vi "ESC_control.vi"(3 "Mode":T5=enum."Run VI", 5 "Traverse line In":T2={"Start X"=0.0, "Start Y"=0.0, "Start Z"=0.0, "End X"=0.0, "End Y"=0.0, "End Z"=0.0, "No. of pts."=0, "Spacing"=enum."Linear", "Filename"=path "", "Tunnel Speed"=0.0, "Averaging time (min)"=0.0, "Extra Commands"="", "Carrier_1 Q (l/min)"=0.0, "Carrier_2 Q (l/min)"=0.0, "Trace Gas Concentration (%)"=0.0, "Specific Arguments"="Source_Live_Control.vi; 1", "Comments"="", "Row No"=0, "Row Type Selector"=enum."Move Traverse Only", "Completion time"="", "Row Duration (mins)"=0.0, "No. of Valid pts."=0, "Meas Setup File"=""} {"Carrier_2 Q (l/min)" format="%#.2f"; "Row Duration (mins)" format="%#.1f"; "Row No" min=0; "Trace Gas Concentration (%)" min=0.0 format="%#_4f"; "Carrier_1 Q (l/min)" format="%#.2f"; "Tunnel Speed" format="%#.2f"; "Start X" format="%#.2f"; "Start Y" format="%#.2f"; "Start Z" format="%#.2f"; "End X" format="%#.2f"; "End Y" format="%#.2f"; "End Z" format="%#.2f"; "Averaging time (min)" min=0.0 format="%#.2f"}) -> (0 "Error Message":string, 1 "Status":T1, 2 "Traverse line Out":T2={"Start X"=0.0, "Start Y"=0.0, "Start Z"=0.0, "End X"=0.0, "End Y"=0.0, "End Z"=0.0, "No. of pts."=0, "Spacing"=enum."Linear", "Filename"=path "", "Tunnel Speed"=0.0, "Averaging time (min)"=0.0, "Extra Commands"="", "Carrier_1 Q (l/min)"=0.0, "Carrier_2 Q (l/min)"=0.0, "Trace Gas Concentration (%)"=0.0, "Specific Arguments"="Source_Live_Control.vi; 1", "Comments"="", "Row No"=0, "Row Type Selector"=enum."Move Traverse Only", "Completion time"="", "Row Duration (mins)"=0.0, "No. of Valid pts."=0, "Meas Setup File"=""} {"Carrier_2 Q (l/min)" format="%#.2f"; "Row Duration (mins)" format="%#.1f"; "Row No" min=0; "Trace Gas Concentration (%)" min=0.0 format="%#_4f"; "Carrier_1 Q (l/min)" format="%#.2f"; "Tunnel Speed" format="%#.2f"; "Start X" format="%#.2f"; "Start Y" format="%#.2f"; "Start Z" format="%#.2f"; "End X" format="%#.2f"; "End Y" format="%#.2f"; "End Z" format="%#.2f"; "Averaging time (min)" min=0.0 format="%#.2f"})   [LabVIEW 2017]
uses:
  Gen Trav/Traverse_cluster.ctl
  Gen Trav/Spacing.ctl
  Controls/Multi_run_mode.ctl
  Controls/User_Specific_mode.ctl
  Gen Trav/Multi_Run_Status.ctl
panel:
  in  "Port":refnum<visa-resource-name>="COM11"
  # "X           Y            Z"
  # "Start"
  # "End"
  # "X           Y            Z"
  # "Start"
  # "End"
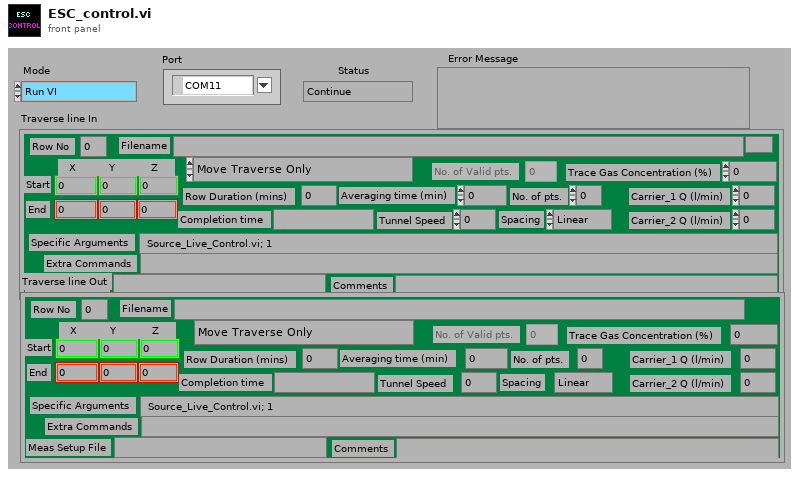
[diagram p1: front panel]
types:
  T1 = typedef "Multi_Run_Status.ctl" = enum16{"Continue", "Continue with Error", "Jump to Next Point", "Jump to Next Row", "Jump To Fall Back", "Terminate Run"}
  T2 = typedef "Traverse_cluster.ctl" = cluster{"Start X":sgl, "Start Y":sgl, "Start Z":sgl, "End X":sgl, "End Y":sgl, "End Z":sgl, "No. of pts.":i32, "Spacing":T3, "Filename":path, "Tunnel Speed":dbl, "Averaging time (min)":dbl, "Extra Commands":string, "Carrier_1 Q (l/min)":dbl, "Carrier_2 Q (l/min)":dbl, "Trace Gas Concentration (%)":dbl, "Specific Arguments":string, "Comments":string, "Row No":i32, "Row Type Selector":T4, "Completion time":string, "Row Duration (mins)":dbl, "No. of Valid pts.":i32, "Meas Setup File":string}
  T3 = typedef "Spacing.ctl" = enum16{"Linear", "Log", "Gauss", "Specified", "N/A"}
  T4 = typedef "Multi_run_mode.ctl" = enum16{"Move Traverse Only", "Set Tunnel Speed Only", "Set Source Only", "Set Measurement Conditions", "Single Measurement", "Vertical Profile", "Lateral Profile", "Longitudinal Profile", "Explore Volume", "Multi-Axis Profile", "Auto Calibrate", "Meas Fast FID Bkgnd", "Check Beam Power", "Scanning Valve Measurement", "Run VI Named:", "Set ADAM Ch", "Wait (minutes)", "Send Message", "Synchronize With:", "Fall Back to this Row", "Turn Off Row Repeating", "Blank Row", "Traverse 3D Volume"}
  T5 = typedef "User_Specific_mode.ctl" = enum16{"Check VI only", "Run VI"}
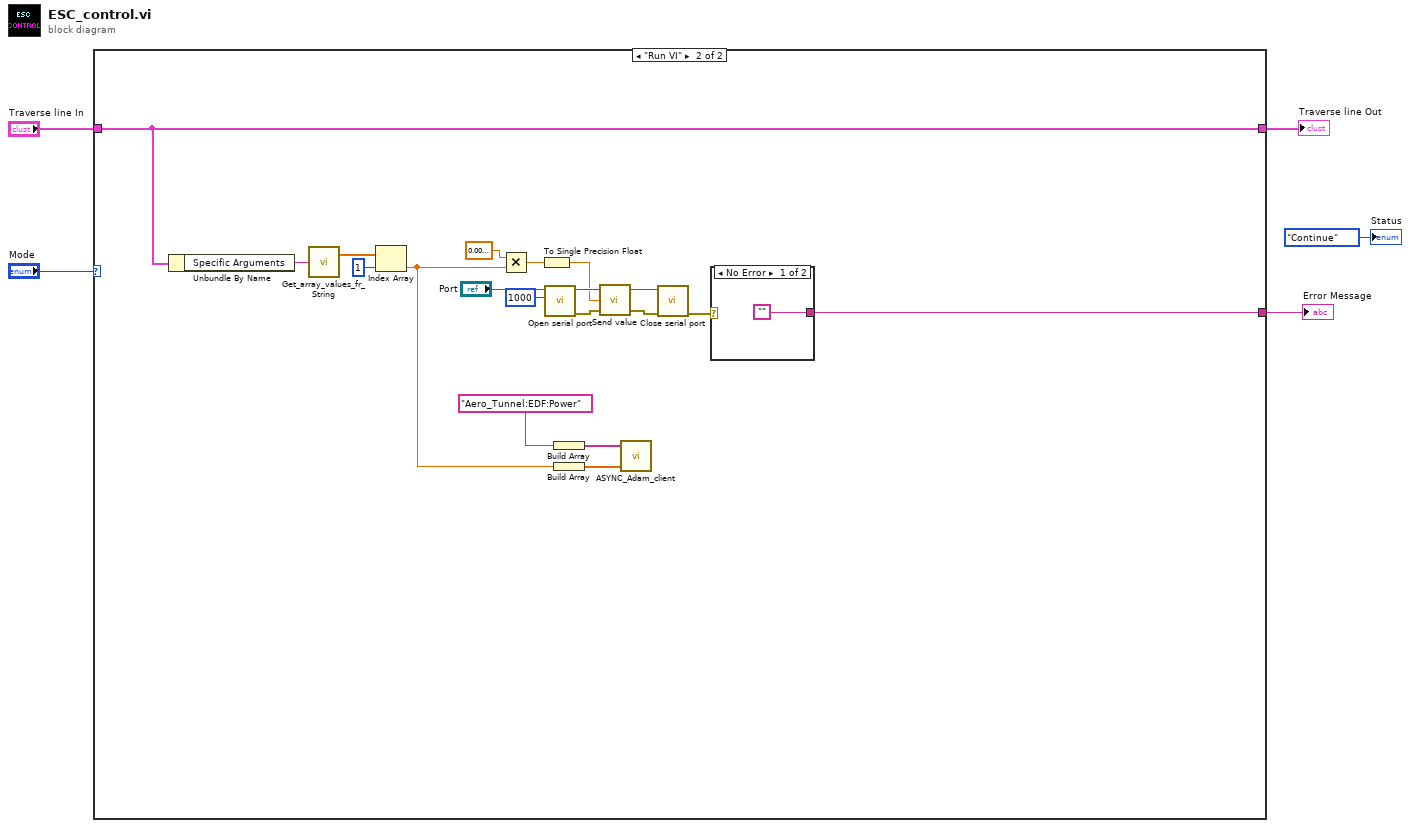
[diagram p0: block diagram]
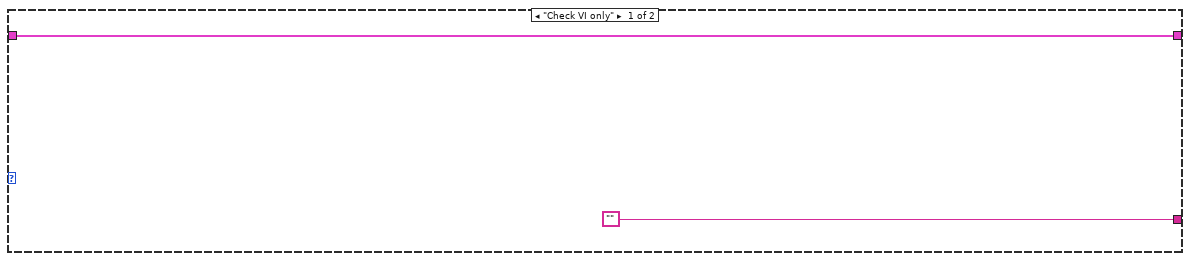
[diagram p2: hidden frame]
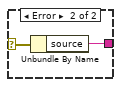
[diagram p3: hidden frame]
diagram:
  n1 = case shown="\"Run VI\"" "Mode" {
    tunnel: "Traverse line In" -> [w7 w26]
    tunnel: [w7 w26] -> w3
    tunnel: ["" w13] -> w2
    frame "Check VI only" {
    }
    frame "Run VI" {
      n2 = Unbundle By Name(w26) -> ("Specific Arguments"=w25:string)
      n3 = call "Get_array_values_fr_String.vi"("String Value"=w25) -> ("Numeric Array"=w24:dbl[])  [unwired: 1 out]
      n4 = Index Array(array=w24, index=1) -> (element=w9:dbl)
      n5 = Multiply(x=0.009999999776482582, y=w9) -> (x*y=w19:dbl)
      n6 = To Single Precision Float(number=w19) -> (single precision float=w14:sgl)
      n7 = call "Open serial port.vi"("timeout (ms)"=u32 1000, "VISA resource name"="Port") -> ("Error out"=w17:errorcluster, "VISA resource name out"=w18:refnum<visa-resource-name>)  [unwired: 8 in]
      n8 = Build Array("Aero_Tunnel:EDF:Power") -> (w10:string[])
      n9 = Build Array(w9) -> (w11:dbl[])
      n10 = call "Send value.vi"("Error In"=w17, "Output (0...1)"=w14, "Port"=w18) -> ("Error Out"=w21:errorcluster, "Port out"=w22:refnum<visa-resource-name>)  [unwired: 1 out]
      n11 = call "ASYNC_Adam_client.vi"("Values"=w11, "Channel Names"=w10) -> ()  [unwired: 1 in, 2 out]
      n12 = call "Close serial port.vi"("Error in"=w21, "VISA resource name"=w22) -> ("Error out"=w12:errorcluster)  [unwired: 9 in]
      n13 = case shown="No Error" w12 {
        selector: w12 -> [_ w28]
        tunnel: ["" w29] -> w13
        frame No Error {
        }
        frame Error {
          n14 = Unbundle By Name(w28) -> ("source"=w29:string)
        }
      }
    }
  }
  "Traverse line Out" <- w3
  "Error Message" <- w2
  "Status" <- Multi_Run_Status."Continue" ("Status")
